vi "loop_period.vi"() -> (0 "t":dbl, 1 "dt":dbl)   [LabVIEW 2021]
uses:
  <vilib>/ptbypt/NI_PtbyPt.lvlib
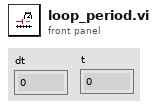
[diagram p1: front panel]
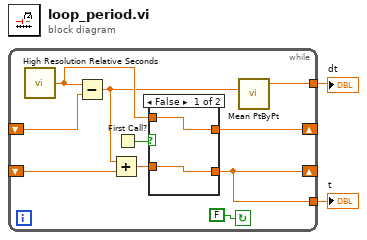
[diagram p0: block diagram]
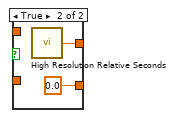
[diagram p2: hidden frame]
diagram:
  n1 = while {
    shift-right: [w10] -> _
    shift-left: _ -> [w12]
    tunnel: [w3] -> w2
    shift-right: [w5] -> _
    shift-left: _ -> [w7]
    tunnel: [w5] -> w1
    stop <- FALSE continue-if-true
    n2 = call <vilib>:"High Resolution Relative Seconds.vi"() -> ("relative seconds"=w9:dbl)
    n3 = Subtract(x=w9, y=w12) -> (x-y=w4:dbl)
    n4 = Add(x=w4, y=w7) -> (x+y=w6:dbl)
    n5 = First Call?() -> (First Call?: T/F=w11:bool)
    n6 = case shown="False" w11 {
      tunnel: [w14 w16] -> w10
      tunnel: w9 -> [w14 _]
      tunnel: [w13 0.0] -> w5
      tunnel: w6 -> [w13 _]
      frame False {
      }
      frame True {
        n7 = call <vilib>:"High Resolution Relative Seconds.vi"() -> ("relative seconds"=w16:dbl)
      }
    }
    n8 = call <vilib>:"Mean PtByPt.vi"("x"=w4) -> ("mean"=w3:dbl)  [unwired: 3 in, 1 out]
  }
  "dt" <- w2
  "t" <- w1
